vi "assignment.vi"() -> ()   [LabVIEW 2024]
panel:
  out "?":bool
  out "?":bool
  out "?":bool
  out "?":bool
  in  "Mile":bool
  in  "Yard":bool
  in  "Feet":bool
  in  "Inch":bool
  in  "stop":bool
  out "Mile":dbl
  out "Yard":dbl
  out "Feet":dbl
  out "Inch":dbl
  in  "Given Value":dbl
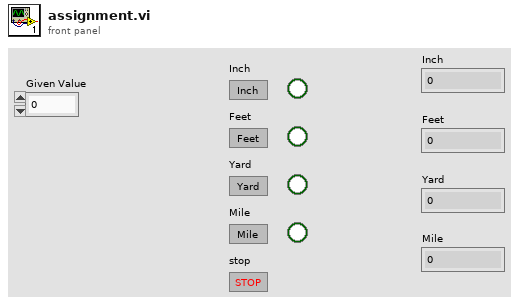
[diagram p1: front panel]
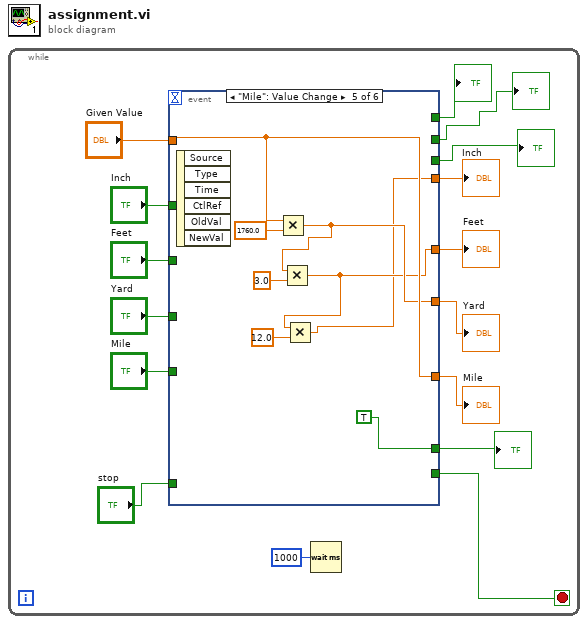
[diagram p0: block diagram]
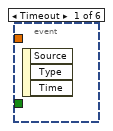
[diagram p2: hidden frame]
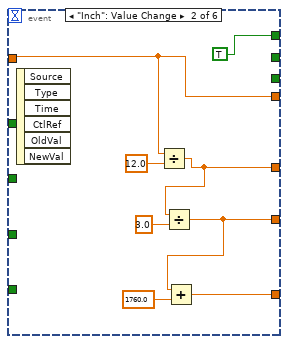
[diagram p3: hidden frame]
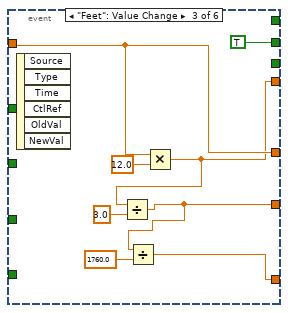
[diagram p4: hidden frame]
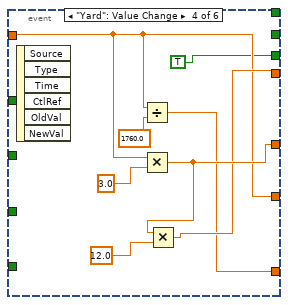
[diagram p5: hidden frame]
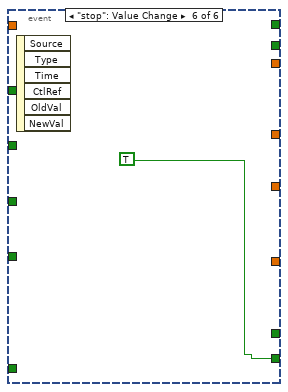
[diagram p6: hidden frame]
diagram:
  n1 = while {
    stop <- w6 stop-if-true
    n2 = event shown="[4] \"Mile\": Value Change" {
      selector: _ -> [_ _ _ _ _ _]
      dyn-events: _ -> [_ _ _ _ _ _]
      timeout: _ -> [_ _ _ _ _ _]
      tunnel: "Given Value" -> [_ w24 w32 w36 w48 _]
      tunnel: "stop" -> [_ _ _ _ _ _]
      tunnel: "Inch" -> [_ _ _ _ _ _]
      tunnel: "Feet" -> [_ _ _ _ _ _]
      tunnel: "Yard" -> [_ _ _ _ _ _]
      tunnel: "Mile" -> [_ _ _ _ _ _]
      tunnel: [_ w24 w30 w37 w42 _] -> w10
      tunnel: [_ w22 w32 w39 w44 _] -> w9
      tunnel: [_ w20 w28 w36 w46 _] -> w8
      tunnel: [_ w18 w26 w34 w48 _] -> w7
      tunnel: [_ _ _ _ _ TRUE] -> w6
      tunnel: [_ TRUE _ _ _ _] -> w4
      tunnel: [_ _ TRUE _ _ _] -> w3
      tunnel: [_ _ _ TRUE _ _] -> w2
      tunnel: [_ _ _ _ TRUE _] -> w1
      event Timeout {
        n3 = event-data() -> ()  [unwired: 1 in, 3 out]
      }
      event "Inch": Value Change {
        n4 = event-data() -> ()  [unwired: 1 in, 6 out]
        n5 = Divide(x=w24, y=12.0) -> (x/y=w22:dbl)
        n6 = Divide(x=w22, y=3.0) -> (x/y=w20:dbl)
        n7 = Add(x=w20, y=1760.0) -> (x+y=w18:dbl)
      }
      event "Feet": Value Change {
        n8 = event-data() -> ()  [unwired: 1 in, 6 out]
        n9 = Multiply(x=w32, y=12.0) -> (x*y=w30:dbl)
        n10 = Divide(x=w30, y=3.0) -> (x/y=w28:dbl)
        n11 = Divide(x=w28, y=1760.0) -> (x/y=w26:dbl)
      }
      event "Yard": Value Change {
        n12 = event-data() -> ()  [unwired: 1 in, 6 out]
        n13 = Divide(x=w36, y=1760.0) -> (x/y=w34:dbl)
        n14 = Multiply(x=w36, y=3.0) -> (x*y=w39:dbl)
        n15 = Multiply(x=w39, y=12.0) -> (x*y=w37:dbl)
      }
      event "Mile": Value Change {
        n16 = event-data() -> ()  [unwired: 1 in, 6 out]
        n17 = Multiply(x=w48, y=1760.0) -> (x*y=w46:dbl)
        n18 = Multiply(x=w46, y=3.0) -> (x*y=w44:dbl)
        n19 = Multiply(x=w44, y=12.0) -> (x*y=w42:dbl)
      }
      event "stop": Value Change {
        n20 = event-data() -> ()  [unwired: 1 in, 6 out]
      }
    }
    "Inch" <- w10
    "Feet" <- w9
    "Yard" <- w8
    "Mile" <- w7
    "?" <- w4
    "?" <- w3
    "?" <- w2
    "?" <- w1
    n21 = Wait (ms)(milliseconds to wait=u32 1000) -> ()  [unwired: 1 out]
  }
